vi "Walk Up to Repository.vi"(8 "error in (no error)":errorcluster, 11 "Build Path":path) -> (0 "error out":errorcluster, 3 "Repository Path":path)   [LabVIEW 2019, in "Git.lvclass"]
uses:
  Git.lvclass
  <vilib>/Utility/error.llb/Error Cluster From Error Code.vi
  <vilib>/ErrorRing/Error Ring.xnode
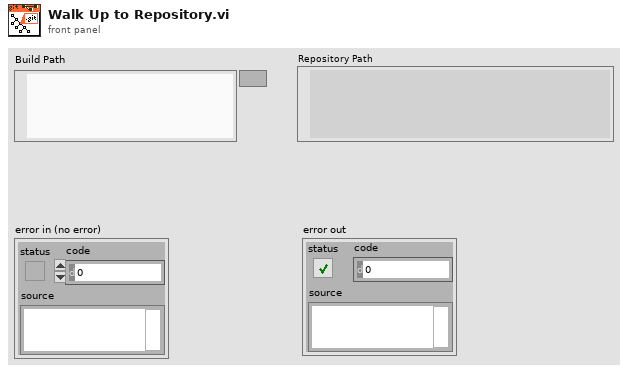
[diagram p1: front panel]
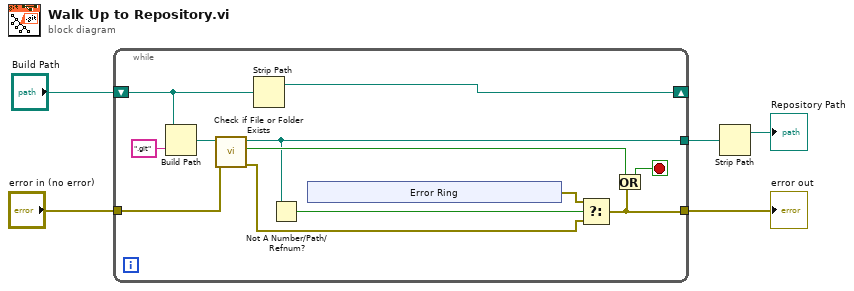
[diagram p0: block diagram]
diagram:
  n1 = while {
    shift-right: [w16] -> _
    shift-left: "Build Path" -> [w15]
    tunnel: [w7] -> w3
    tunnel: "error in (no error)" -> [w6]
    tunnel: [w8] -> w2
    stop <- w11 stop-if-true
    n2 = Build Path(base path=w15, name or relative path=".git") -> (appended path=w14:path)
    n3 = call <vilib>:"Check if File or Folder Exists.vi"("error in (no error)"=w6, "path"=w14) -> ("error out"=w9:errorcluster, "file or folder exists?"=w12:bool, "dup path"=w7:path)  [unwired: 7 in]
    n4 = Strip Path(path=w15) -> (stripped path=w16:path)  [unwired: 1 out]
    n5 = Not A Number/Path/Refnum?(number/path/refnum=w7) -> (NaN/Path/Refnum?=w13:bool)
    n6 = xnode "Error Ring"() -> ("error out"=w10:errorcluster)
    n7 = Select(t=w10, s=w13, f=w9) -> (s? t:f=w8:errorcluster)
    n8 = Or(x=w12, y=w8) -> (x .or. y?=w11:bool)
  }
  "error out" <- w2
  n9 = Strip Path(path=w3) -> (stripped path=→"Repository Path":path)  [unwired: 1 out]
